vi "TCPCommunication.vi"(0 "Send Data":string, 11 "error in (no error)":errorcluster, 13 "Selector":T1(ring)) -> (4 "Recieve data":string, 15 "error out":errorcluster)   [LabVIEW 2014]
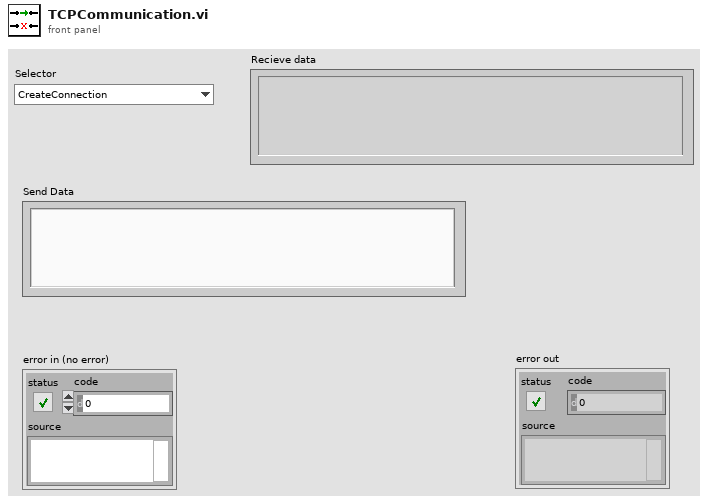
[diagram p1: front panel]
types:
  T1 = enum16{"CreateConnection", "WriteData", "ReadData", "CloseConnection"}
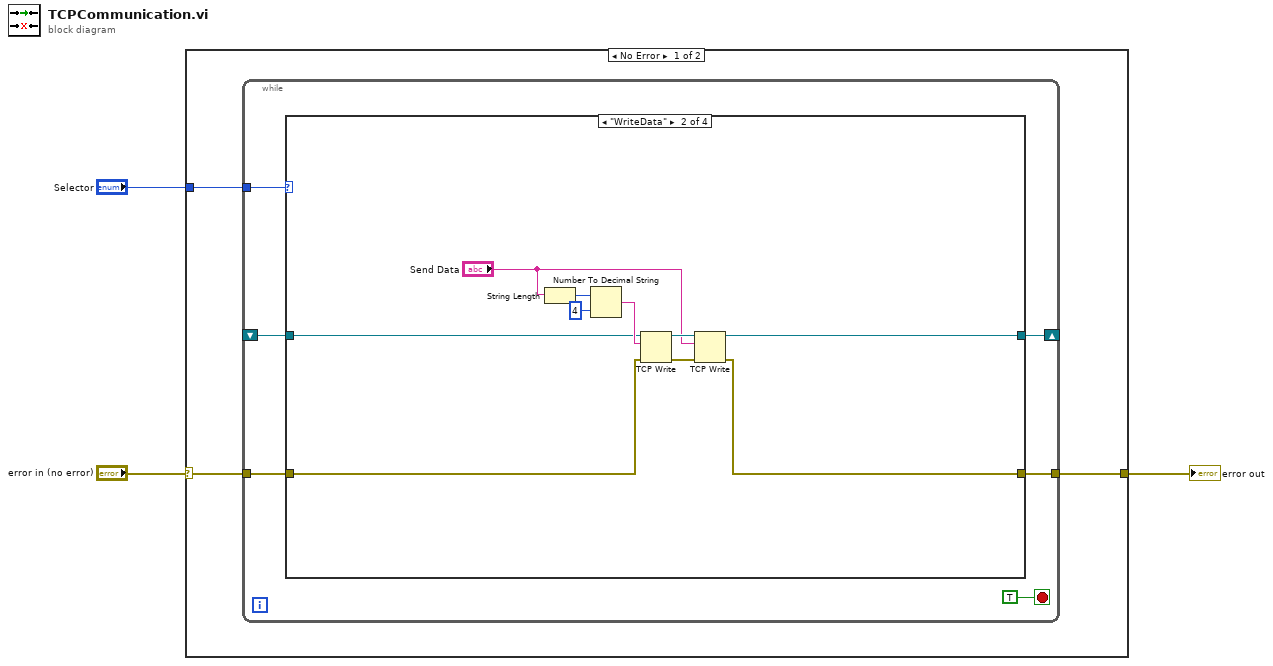
[diagram p0: block diagram]
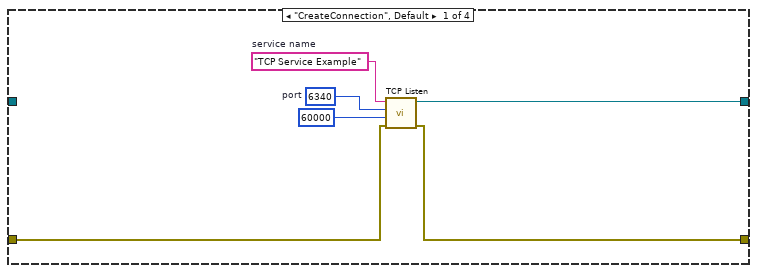
[diagram p2: hidden frame]
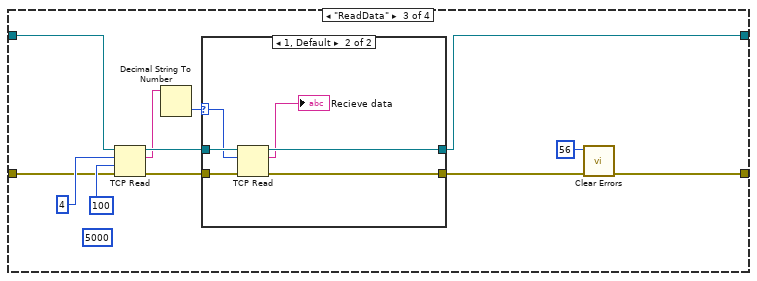
[diagram p3: hidden frame]
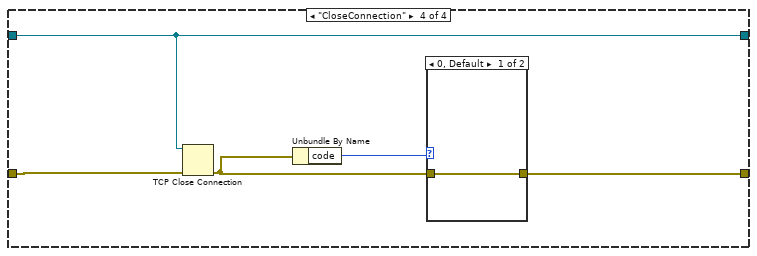
[diagram p5: hidden frame]
diagram:
  n1 = case shown="No Error" "error in (no error)" {
    selector: "error in (no error)" -> [w5 w55]
    tunnel: "Selector" -> [w6 _]
    tunnel: [w4 w55] -> w1
    frame No Error {
      n2 = while {
        tunnel: w6 -> [w11]
        tunnel: w5 -> [w10]
        tunnel: [w9] -> w4
        shift-right: [w8] -> _
        shift-left: _ -> [w7]
        stop <- TRUE stop-if-true
        n3 = case shown="\"WriteData\"" w11 {
          tunnel: w10 -> [w15 w22 w32 w53]
          tunnel: [w14 w19 w31 w50] -> w9
          tunnel: [w13 w20 w30 w49] -> w8
          tunnel: w7 -> [_ w21 w29 w49]
          frame "CreateConnection", Default {
            w16 = u16 6340  # port
            w18 = "TCP Service Example"  # service name
            n4 = call <vilib>:"TCP Listen.vi"("error in (no error)"=w15, "timeout ms (wait forever: -1)"=60000, "port"=w16, "service name"=w18) -> ("error out"=w14:errorcluster, "connection ID"=w13:refnum<k5>)  [unwired: 3 in, 3 out]
          }
          frame "WriteData" {
            n5 = String Length(string="Send Data") -> (length=w25:i32)
            n6 = Number To Decimal String(number=w25, width (-)=i16 4) -> (decimal integer string=w23:string)
            n7 = TCP Write(connection ID=w21, data in=w23, error in (no error)=w22) -> (connection ID out=w28:refnum<k5>, error out=w27:errorcluster)  [unwired: 2 out]
            n8 = TCP Write(connection ID=w28, data in="Send Data", error in (no error)=w27) -> (connection ID out=w20:refnum<k5>, error out=w19:errorcluster)  [unwired: 2 out]
          }
          frame "ReadData" {
            (unwired) 5000 ("timeout ms (25000)")
            n9 = TCP Read(connection ID=w29, bytes to read=4, error in (no error)=w32, 9:100 ("timeout ms (25000)")) -> (connection ID out=w38:refnum<k5>, data out=w34:string, error out=w37:errorcluster)  [unwired: 1 in]
            n10 = Decimal String To Number(string=w34) -> (number=w33:i32)  [unwired: 2 in, 1 out]
            n11 = case shown="1, Default" w33 {
              selector: w33 -> [_ w44]
              tunnel: w38 -> [w41 w48]
              tunnel: w37 -> [w42 w47]
              tunnel: [w42 w45] -> w36
              tunnel: [w41 w46] -> w30
              frame 0 {
              }
              frame 1, Default {
                n12 = TCP Read(connection ID=w48, bytes to read=w44, error in (no error)=w47) -> (connection ID out=w46:refnum<k5>, data out=→"Recieve data":string, error out=w45:errorcluster)  [unwired: 2 in]
              }
            }
            n13 = call <vilib>:"Clear Errors.vi"("error in (no error)"=w36, "specific error code to clear (0: all)"=56) -> ("error out"=w31:errorcluster)  [unwired: 4 in, 1 out]
          }
          frame "CloseConnection" {
            n14 = TCP Close Connection(connection ID=w49, error in (no error)=w53) -> (error out=w51:errorcluster)  [unwired: 1 in, 1 out]
            n15 = Unbundle By Name(w51) -> ("code"=w52:i32)
            n16 = case shown="0, Default" w52 {
              tunnel: [w54 _] -> w50
              tunnel: w51 -> [w54 _]
              frame 0, Default {
              }
              frame 62, 64, 66 {
              }
            }
          }
        }
      }
    }
    frame Error {
    }
  }
  "error out" <- w1
